vi "Str2Num.vi"(2 "str_data":string) -> (7 "arr_values":u64[](array[numeric]))   [LabVIEW 2022 SP3]
uses:
  <vilib>/regexp/Match Regular Expression.xnode
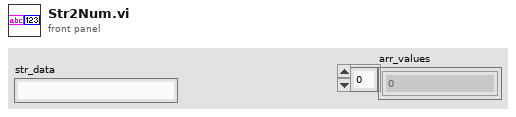
[diagram p1: front panel]
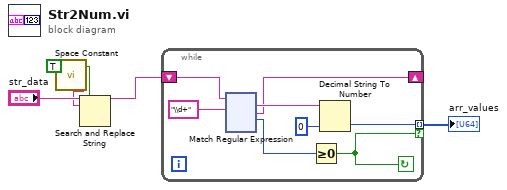
[diagram p0: block diagram]
diagram:
  n1 = call <vilib>:"Space Constant.vi"() -> ("String"=w2:string)
  n2 = Search and Replace String(replace all?=TRUE ("replace all? (F)"), input string="str_data", search string=w2) -> (result string=w4:string)  [unwired: 5 in, 3 out]
  n3 = while {
    tunnel: [w10] -> w5 mode=indexing if=w9
    shift-right: [w6] -> _
    shift-left: w4 -> [w13]
    stop <- w9 continue-if-true
    n4 = xnode "Match Regular Expression"("input string"=w13, "regular expression"="\\d+") -> ("whole match"=w7:string, "after match"=w6:string, "offset past match"=w8:i32)  [unwired: 4 in, 2 out]
    n5 = Greater Or Equal To 0?(x=w8) -> (x >= 0?=w9:bool)
    n6 = Decimal String To Number(string=w7, default (0L)=u64 0) -> (number=w10:u64)  [unwired: 1 in, 1 out]
  }
  "arr_values" <- w5
